vi "Get Dependencies.vi"(0 "vi path":path, 11 "error in":errorcluster) -> (4 "existing dependencies":path[](array[path]), 15 "error out":errorcluster)   [LabVIEW 2021, in "Multiple Converter.lvlib"]
uses:
  Multiple Converter.lvlib
  Converter Reusables/Converter Reusables.lvlib
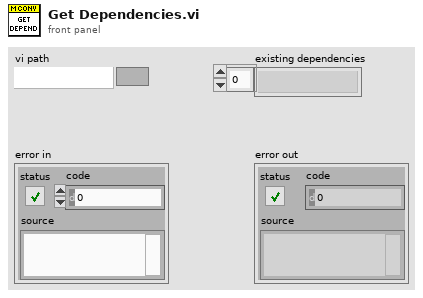
[diagram p1: front panel]
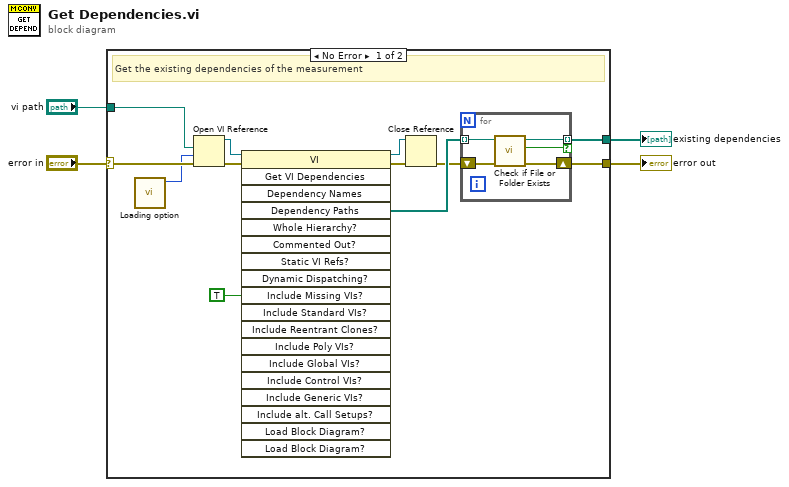
[diagram p0: block diagram]
diagram:
  n1 = case shown="No Error" "error in" {
    selector: "error in" -> [w7 w22]
    tunnel: [w16 _] -> w4
    tunnel: [w6 w22] -> w3
    tunnel: "vi path" -> [w8 _]
    frame No Error {
      # "Get the existing dependencies of the measurement"
      n2 = call "Loading option.vi"() -> ("options"=w5:i32)  [unwired: 11 in]
      n3 = Open VI Reference(vi path=w8, options=w5, error in (no error)=w7) -> (vi reference=w9:refnum<vi>, error out=w10:errorcluster)  [unwired: 3 in]
      n4 = invoke class="VI" method="Get VI Dependencies"(reference=w9, error in=w10, "Include Missing VIs?"=TRUE ("Include Missing Items?")) -> (reference out=w12:refnum<vi>, error out=w11:errorcluster, "Dependency Paths"=w15:path[])  [unwired: 16 in, 16 out]
      n5 = Close Reference(reference=w12, error in (no error)=w11) -> (error out=w14:errorcluster)
      n6 = for {
        tunnel: w15 -> [w20] mode=indexing
        tunnel: [w19] -> w16 mode=indexing if=w18
        shift-right: [w17] -> w6
        shift-left: w14 -> [w21]
        n7 = call <vilib>:"Check if File or Folder Exists.vi"("error in (no error)"=w21, "path"=w20) -> ("error out"=w17:errorcluster, "file or folder exists?"=w18:bool, "dup path"=w19:path)  [unwired: 7 in]
      }
    }
    frame Error {
    }
  }
  "existing dependencies" <- w4
  "error out" <- w3
